vi "Initiate.vi"(8 "error in":errorcluster, 11 "Configuration filepath":string="C:\\Program Files\\cronologic\\HPTDC8-PCI\\apps\\global.cfg") -> (0 "error out":errorcluster, 2 "Success?":bool, 3 "TDCManager":T1)   [LabVIEW 2016, in "HPTDC Driver Library.lvlib"]
uses:
  HPTDC Driver Library.lvlib
  Typedefs/TDCManager.ctl
  C:/Users/CRT Controller/CRTC Labview Application/Source/HPTDC Driver Library Folder/Library files/hptdc_net4_3.7.0_x64.dll
  hptdc_net4_3.7.0_x64.dll
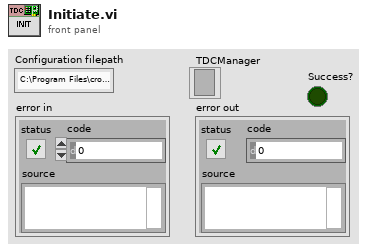
[diagram p1: front panel]
types:
  T1 = typedef "HPTDC Driver Library.lvlib/TDCManager.ctl" = refnum<k24>
  T2 = typedef "Semaphore RefNum" = refnum<k1>
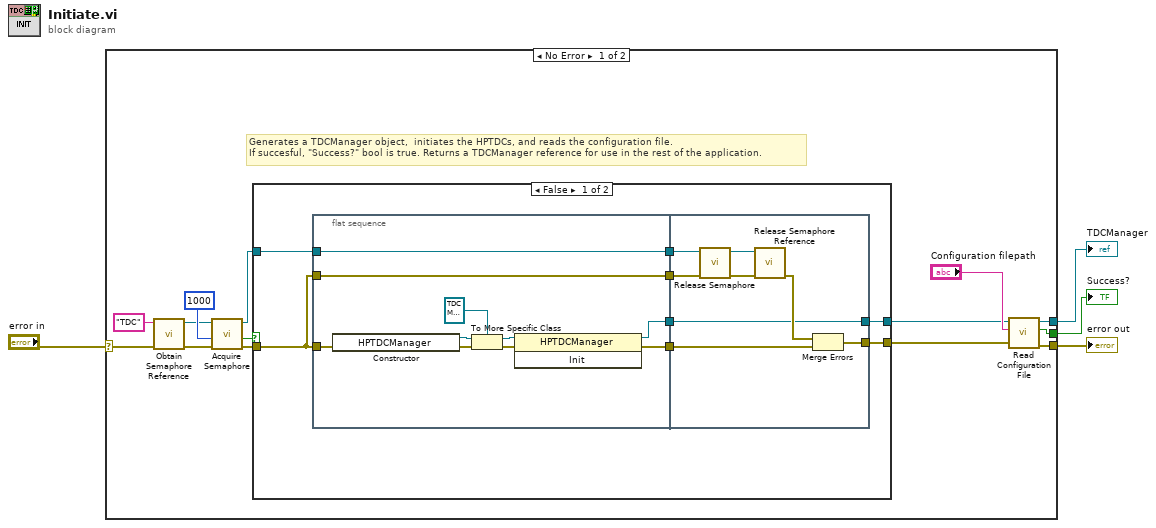
[diagram p0: block diagram]
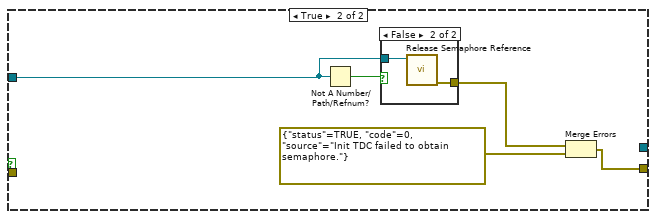
[diagram p2: hidden frame]
diagram:
  n1 = case shown="No Error" "error in" {
    selector: "error in" -> [w5 w52]
    tunnel: [w17 _] -> w4
    tunnel: [w16 w52] -> w3
    tunnel: [w15 _] -> w2
    frame No Error {
      # "Generates a TDCManager object,  initiates the HPTDCs, and reads the configuration file.\nIf succesful, \"Success?\" bool is true. Returns a TDCManager reference for use in the rest of the application."
      n2 = call <vilib>:"Obtain Semaphore Reference.vi"("error in (no error)"=w5, "name (unnamed)"="TDC") -> ("error out"=w12:errorcluster, "semaphore"=w13:T2)  [unwired: 3 in, 1 out]
      n3 = call <vilib>:"Acquire Semaphore.vi"("error in (no error)"=w12, "ms timeout (-1)"=1000, "semaphore"=w13) -> ("error out"=w9:errorcluster, "timed out"=w10:bool, "semaphore out"=w8:T2)  [unwired: 2 in]
      n4 = case shown="False" w10 {
        tunnel: w9 -> [w24 _]
        tunnel: w8 -> [w22 w45]
        tunnel: [w19 _] -> w6
        tunnel: [w21 w47] -> w7
        frame False {
          n5 = flat-sequence {
            tunnel: w24 -> [w29]
            tunnel: [w28] -> w26
            tunnel: w24 -> [w36]
            tunnel: [w36] -> w25
            tunnel: [w35] -> w23
            tunnel: w22 -> [w35]
            tunnel: [w27] -> w20
            tunnel: w26 -> [w44]
            tunnel: w25 -> [w41]
            tunnel: w23 -> [w39]
            tunnel: [w38] -> w21
            tunnel: [w37] -> w19
            tunnel: w20 -> [w37]
            frame #0 {
              n6 = constructor class="HPTDCManager"(error in=w29) -> (reference out=w32:refnum<k24>, error out=w34:errorcluster)  [unwired: 2 in, 1 out]
              n7 = To More Specific Class(target class=T1 refnum ("TDCManager"), reference=w32, error in=w34) -> (specific class reference=w31:T1, error out=w33:errorcluster)
              n8 = invoke class="HPTDCManager" method="Init"(reference=w31, error in=w33) -> (reference out=w27:T1, error out=w28:errorcluster)  [unwired: 1 in, 1 out]
            }
            frame #1 {
              n9 = call <vilib>:"Release Semaphore.vi"("error in (no error)"=w41, "semaphore"=w39) -> ("error out"=w42:errorcluster, "semaphore out"=w43:T2)  [unwired: 4 in]
              n10 = call <vilib>:"Release Semaphore Reference.vi"("error in (no error)"=w42, "semaphore"=w43) -> ("error out"=w40:errorcluster)  [unwired: 8 in, 1 out]
              n11 = Merge Errors(w40, w44) -> (w38:errorcluster)
            }
          }
        }
        frame True {
          n12 = Not A Number/Path/Refnum?(number/path/refnum=w45) -> (NaN/Path/Refnum?=w49:bool)
          n13 = case shown="False" w49 {
            tunnel: [_ w51] -> w46
            tunnel: w45 -> [_ w50]
            frame True {
            }
            frame False {
              n14 = call <vilib>:"Release Semaphore Reference.vi"("semaphore"=w50) -> ("error out"=w51:errorcluster)  [unwired: 9 in, 1 out]
            }
          }
          n15 = Merge Errors(w46, errorcluster {"status"=TRUE, "code"=0, "source"="Init TDC failed to obtain semaphore."} ("error out")) -> (w47:errorcluster)
        }
      }
      n16 = call "Read Configuration File.vi"("error in (no error)"=w7, "Configuration filepath"="Configuration filepath", "TDCManager"=w6) -> ("error out"=w16:errorcluster, "Success?"=w17:bool, "TDCManager"=w15:T1)  [unwired: 6 in]
    }
    frame Error {
    }
  }
  "error out" <- w3
  "Success?" <- w4
  "TDCManager" <- w2
